vi "HAL-AI.vi"(7 "Name(\"\" to use uuid)":string="CSM-Module") -> ()   [LabVIEW 2020]
doc: "------------- lvcsm -------------\n[CSMStates]\nItem 0 = \"Idle\"\nItem 1 = \"CSM Documentation\"\nItem 2 = \"Error Handler\"\nItem 3 = \"VI Reference\"\nItem 4 = \"Critical Error\"\nItem 5 = \"Target Busy Error\"\nItem 6 = \"Target Timeout Error\"\nItem 7 = \"Target Error\"\nItem 8 = \"Async Response\"\nItem 9 = \"Response\"\nItem 10 = \"Async Message Posted\"\nItem 11 = \"Initialize Core Data\"\nItem 12 = \"Exit\"\nItem 13 = \"Data: Initialize\"\nItem 14 = \"Data: Get Configuration\"\nItem 15 = \"Data: Get Internal Data\"\nItem 16 = \"Data: Set Configuration\"\nItem 17 = \"Data: Update Indicators\"\nItem 18 = \"Data: Cleanup\"\nItem 19 = \"Macro: Initialize\"\nItem 20 = \"Macro: Exit\"\nItem 21 = \"Channels\"\nItem 22 = \"read\"\nItem 23 = \"read(massdata)\"\nItem 24 = \"read all\"\nItem 25 = \"DoSth: DoA\"\nItem 26 = \"DoSth: DoB\"\n\n[CSMStatus]\nItem 0 = \"Error Occurred@Error Handler\""
uses:
  4e85c3fb-ef85-4e26-a42c-c5beb394b70a.vi
  3806dceb-3f37-4f57-9f18-971811feca89.vi
  3ab58302-ba21-4fa6-a4e6-5e0190e36a76.vi
  c8f15f2d-01d5-4330-b5b0-2e0c665b45aa.vi
  a8188fcd-c635-40c0-88bb-da73c8fc0970.vi
  2d894bb3-d511-4c50-a434-1d8b5ddcf511.vi
  3a3714ae-08be-45b6-9f70-6e503687bd9b.vi
  0b2eaf5c-92e0-4609-89e4-060a3e7ae5c6.vi
  e9c7e813-d0b7-45e0-ac3a-d1de35bf1555.vi
  <userlib>/_NEVSTOP/Communicable State Machine(CSM)/_Support/Common/Format Timestamp.vi
  <userlib>/_NEVSTOP/Communicable State Machine(CSM)/AdvanceAPI/CSM - Revert Arguments-Safe String.vi
  <userlib>/_NEVSTOP/Communicable State Machine(CSM)/AdvanceAPI/CSM - Make String Arguments Safe.vi
  <userlib>/_NEVSTOP/Communicable State Machine(CSM)/AdvanceAPI/CSM - Break Down Multiple States String.vi
  <userlib>/_NEVSTOP/Communicable State Machine(CSM)/AdvanceAPI/CSM - Compact Multiple States.vi
  <userlib>/_NEVSTOP/Communicable State Machine(CSM)/AdvanceAPI/CSM - Keywords.vi
  <userlib>/_NEVSTOP/Communicable State Machine(CSM)/_Shared/Trim Single-line Text.vi
  <userlib>/_NEVSTOP/Communicable State Machine(CSM)/addons/API-String-Arugments-Support/_Support/Query Data as API String Arguments(variant).vi
  <userlib>/_NEVSTOP/Communicable State Machine(CSM)/addons/API-String-Arugments-Support/_Support/Convert API String Arguments to Data(variant).vi
  <userlib>/_NEVSTOP/Communicable State Machine(CSM)/addons/API-String-Arugments-Support/_Support/Data To API String Arguments.vi
  <userlib>/_NEVSTOP/Communicable State Machine(CSM)/addons/MassData-Parameter/_support/FGV-MassData(lvlibp).vi
  <userlib>/_NEVSTOP/Communicable State Machine(CSM)/Communicable State Machine.lvlib
panel:
  out "Error Occurred":errorcluster
  out "State History":string
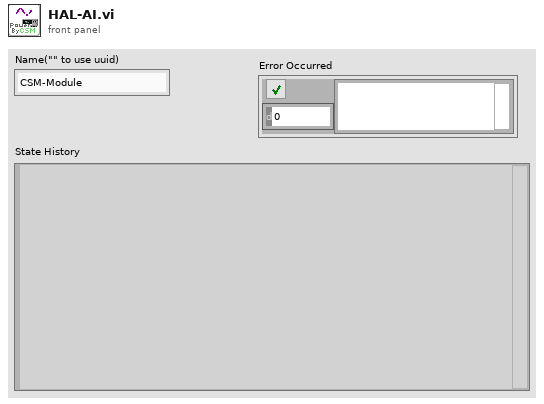
[diagram p1: front panel]
types:
  T1 = enum32{"Invalid", "Standard", "Closed", "Hidden", "Minimized", "Maximized"}
  T2 = enum32{"invalid app kind", "Development System", "Run Time System", "Student Edition", "Embedded LabVIEW", "Evaluation", "Custom"}
  T3 = typedef "Communicable State Machine.lvlib/_CSM_Response Source Message.ctl" = cluster{"‘State":string, "’Arguments":string, "’Error":errorcluster}
  T4 = cluster{"Current VI Reference":refnum<vi>, "Close Panel on Exit?":bool}
  T5 = cluster{"Core":cluster{"Current VI Reference":refnum<vi>, "Close Panel on Exit?":bool}, "Your Boolean data":bool, "Channels":string[]}
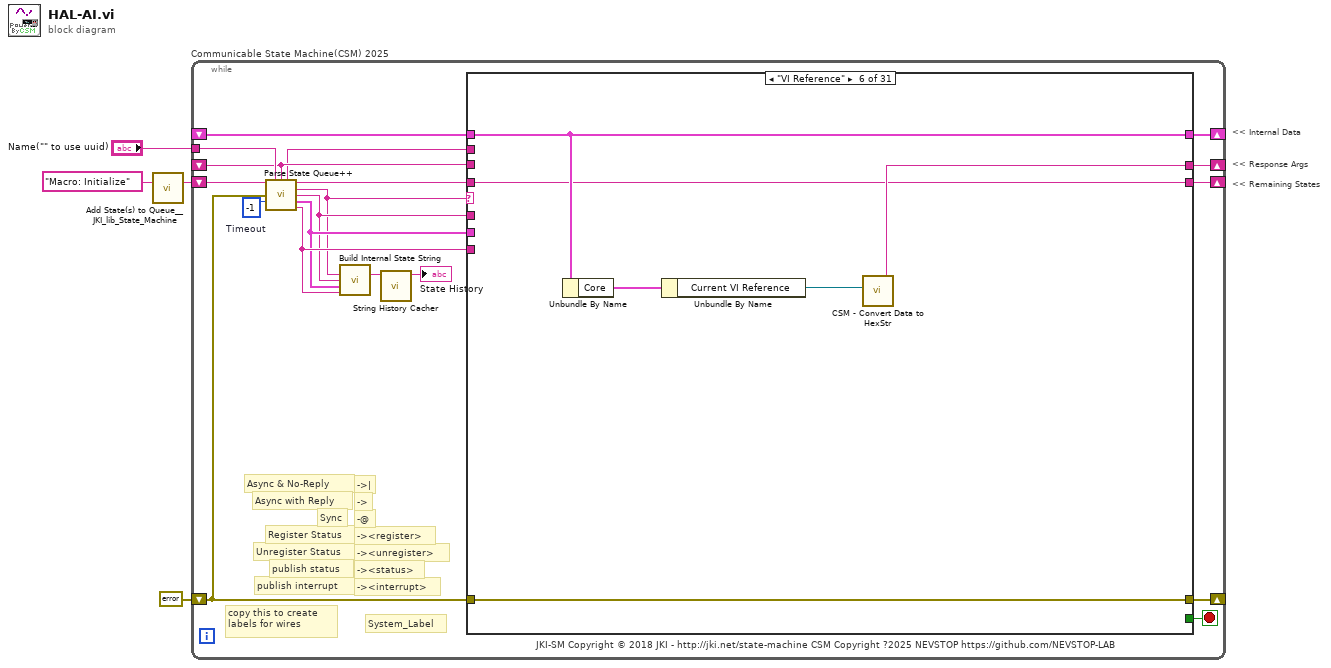
[diagram p0: block diagram]
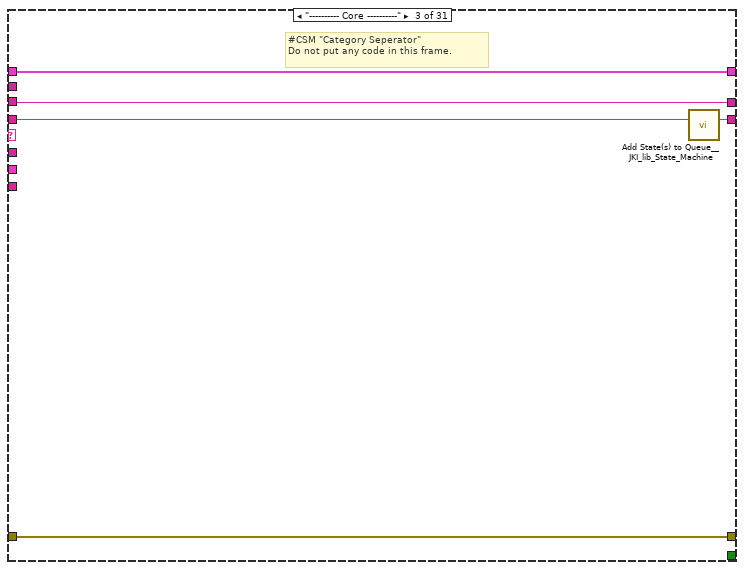
[diagram p4: hidden frame]
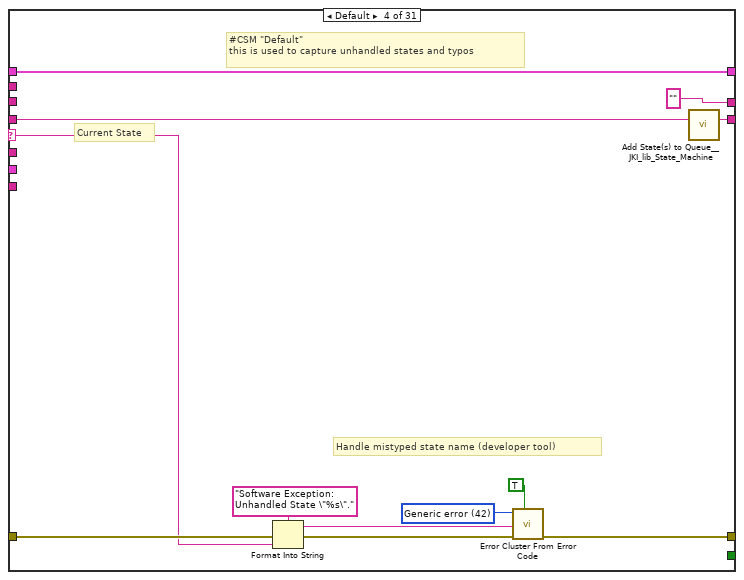
[diagram p5: hidden frame]
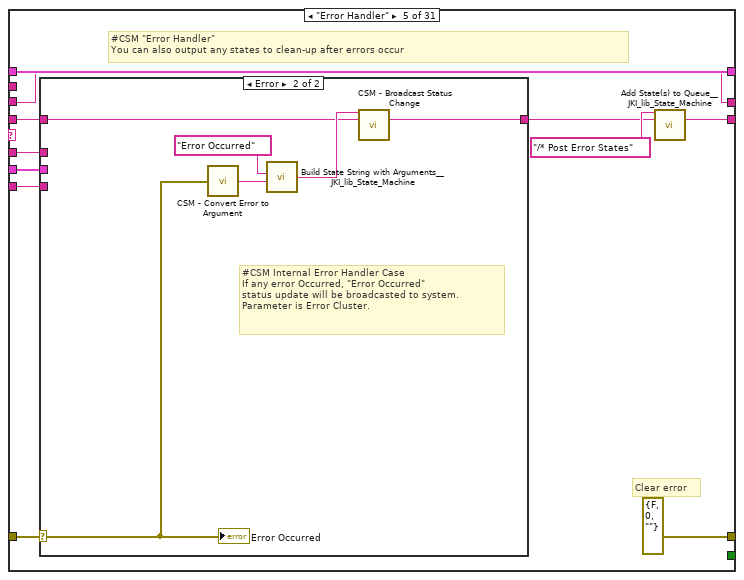
[diagram p6: hidden frame]
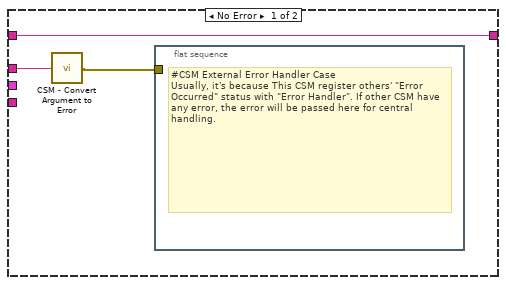
[diagram p7: hidden frame]
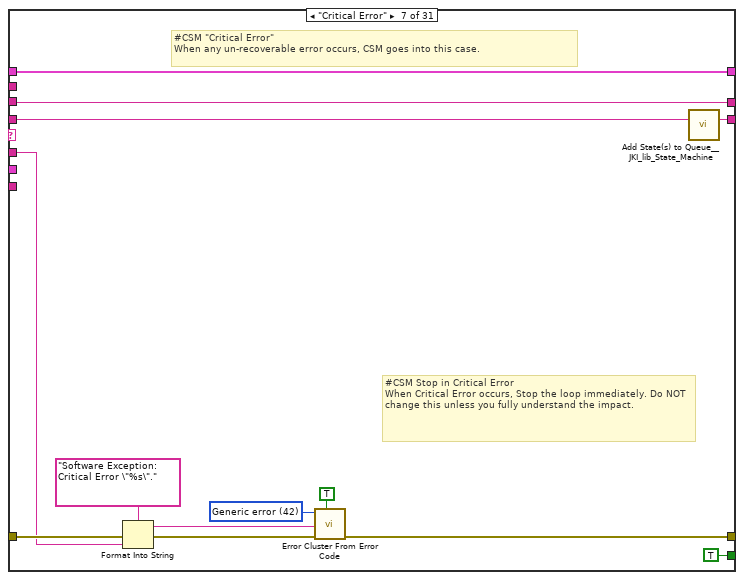
[diagram p8: hidden frame]
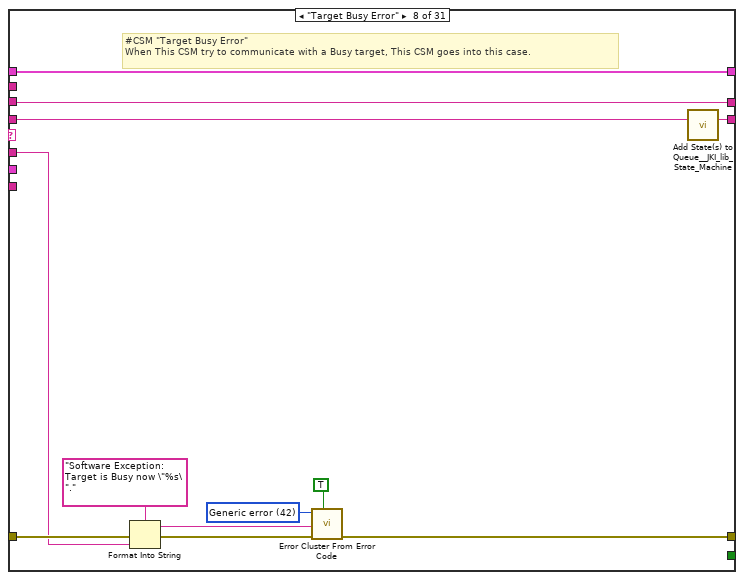
[diagram p9: hidden frame]
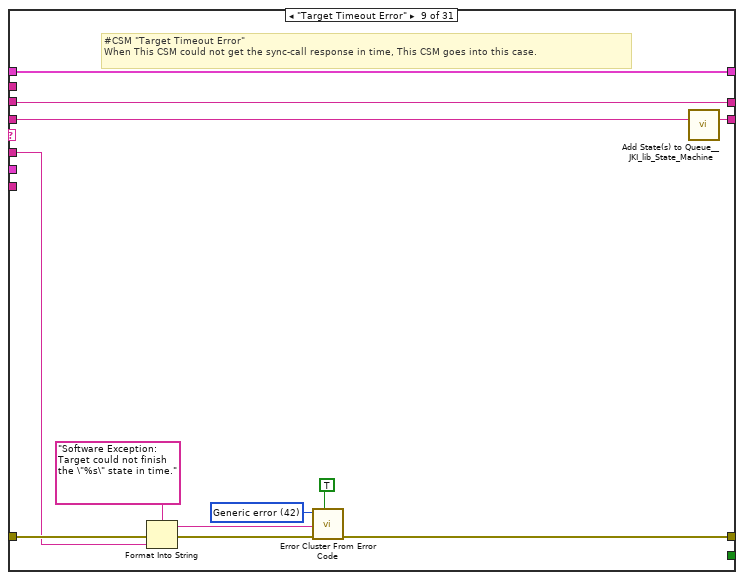
[diagram p10: hidden frame]
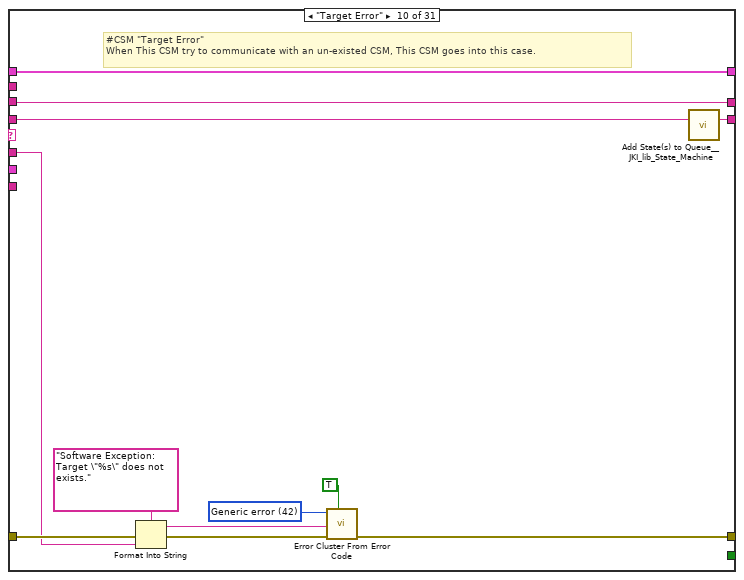
[diagram p11: hidden frame]
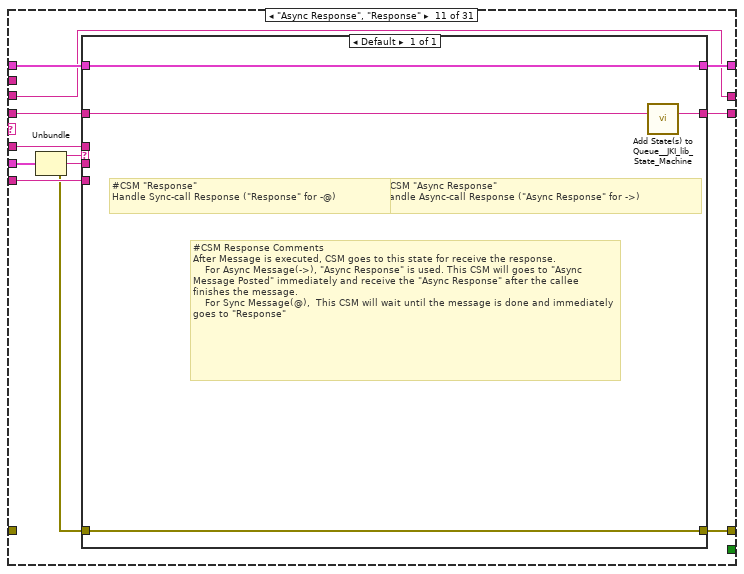
[diagram p12: hidden frame]
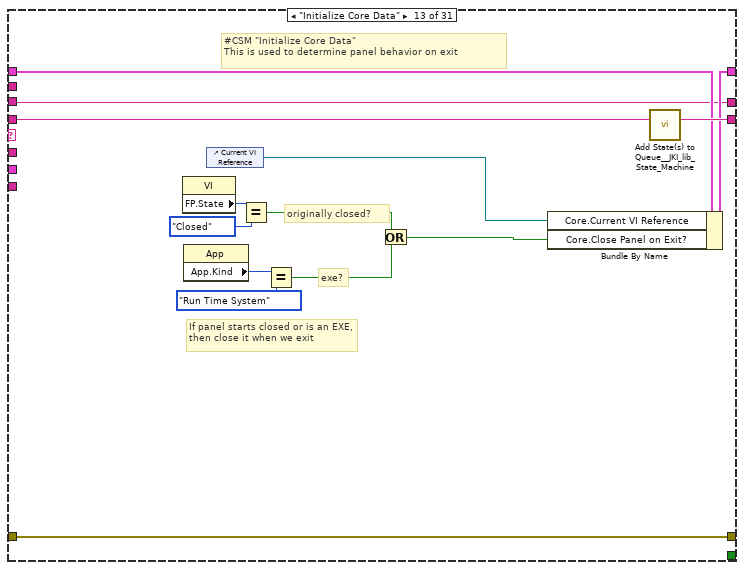
[diagram p14: hidden frame]
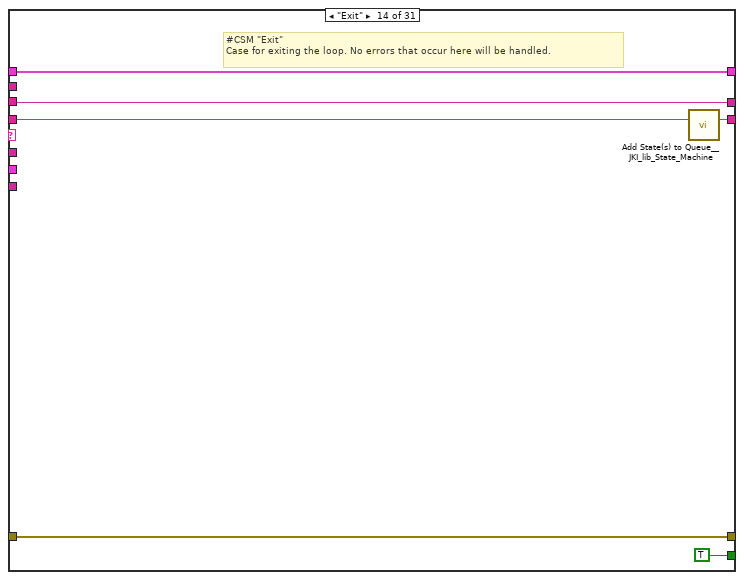
[diagram p15: hidden frame]
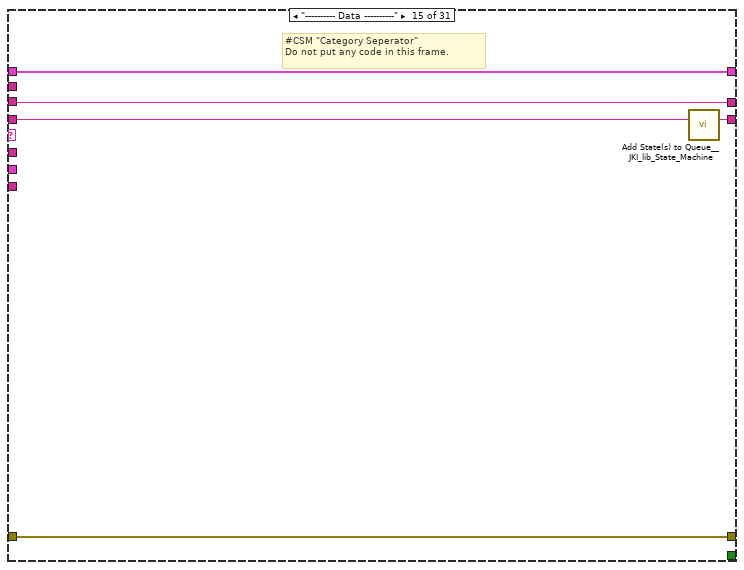
[diagram p16: hidden frame]
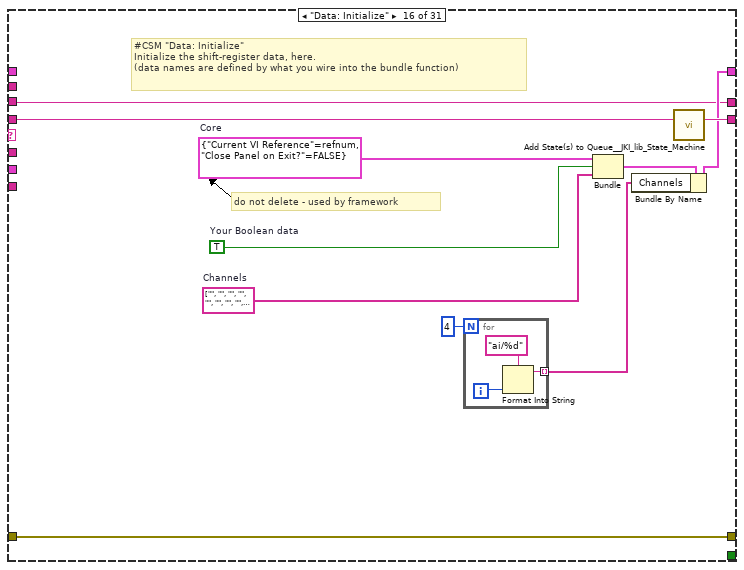
[diagram p17: hidden frame]
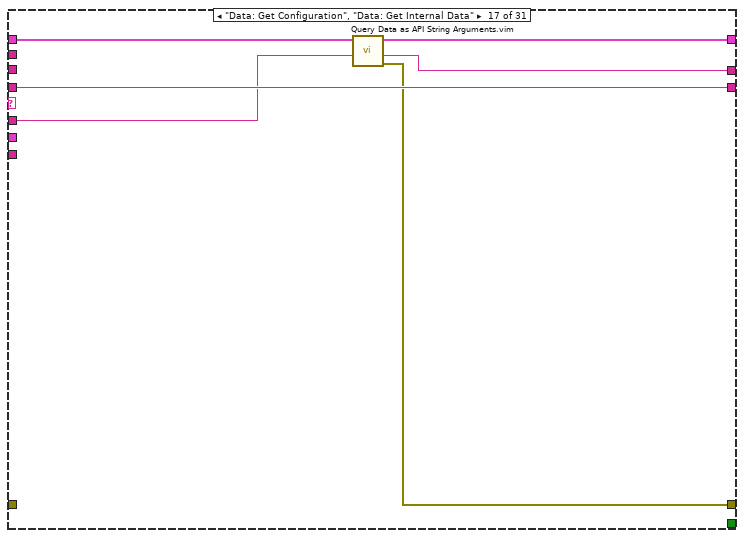
[diagram p18: hidden frame]
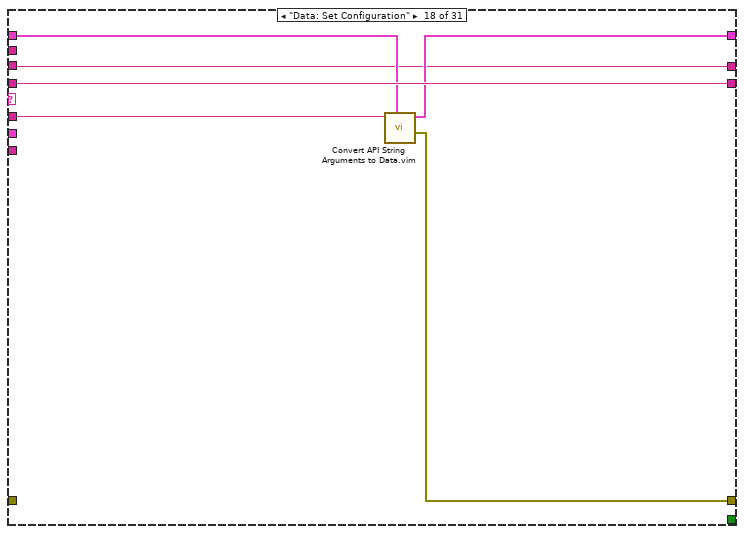
[diagram p19: hidden frame]
diagram:
  # "<< Internal Data"
  # "<< Response Args"
  # "<< Remaining States"
  n1 = call <vilib>:"Add State(s) to Queue__JKI_lib_State_Machine.vi"("State(s) in (\"\")"="Macro: Initialize" ("Init States(\"Macro: Initialize\")")) -> ("States Out"=w3:string)  [unwired: 14 in]
  n2 = while "Communicable State Machine(CSM) 2025" {
    shift-right: [w18] -> _
    shift-left: _ -> [w17]
    shift-right: [w21] -> _
    shift-left: errorcluster {"status"=FALSE, "code"=0, "source"=""} ("error out") -> [w5]
    shift-right: [w20] -> _
    shift-left: w3 -> [w22]
    tunnel: "Name(\"\" to use uuid)" -> [w14]
    shift-right: [w15] -> _
    shift-left: _ -> [w7]
    stop <- w19 stop-if-true
    w16 = -1  # Timeout
    # "copy this to create labels for wires"
    # "System_Label"
    # "-><interrupt>"
    # "-><status>"
    # "-><unregister>"
    # "-><register>"
    # "-@"
    # "->"
    # "->|"
    # "publish interrupt"
    # "publish status"
    # "Unregister Status"
    # "Register Status"
    # "Sync"
    # "Async with Reply"
    # "Async & No-Reply"
    # "JKI-SM Copyright © 2018 JKI - http://jki.net/state-machine CSM Copyright ?2025 NEVSTOP https://github.com/NEVSTOP-LAB"
    n3 = call <userlib>:"Parse State Queue++.vi"("State Queue"=w22, "Name (\"\" to Use UUID)"=w14, "Response Arguments"=w7, "Previous Error"=w5, "Dequeue (1 ms)"=w16) -> ("Name Used"=w6:string, "Remaining States"=w23:string, "Current State"=w8:string, "Arguments"=w9:string, "Additional Information"=w10:T3, "Source CSM"=w11:string)  [unwired: 5 in]
    n4 = call <userlib>:"Build Internal State String.vi"("State"=w8, "Arguments (\"\")"=w9, "Additional Information"=w10, "Source (\"\")"=w11) -> ("State With Arguments"=w12:string)  [unwired: 11 in]
    n5 = call <userlib>:"String History Cacher.vi"("String"=w12) -> ("String Cache"=→"State History":string)  [unwired: 10 in]
    n6 = case shown="\"VI Reference\"" w8 {
      selector: w8 -> [_ _ _ w38 _ _ _ _ _ _ _ _ _ _ _ _ _ _ _ _ _ _ _ _ _ _ _ _ _ _ _]
      tunnel: w23 -> [w25 w30 w36 w42 w53 w70 w81 w94 w106 w118 w129 w142 w157 w163 w168 w179 w188 w194 w197 w205 w210 w216 w222 w225 w230 w250 w273 w291 w300 w305 w310]
      tunnel: w9 -> [_ _ _ _ w52 _ w77 w90 w102 w114 w128 _ _ _ _ _ w183 w193 _ _ _ _ _ _ _ w249 w272 w290 _ _ _]
      tunnel: w17 -> [w26 w29 w33 w40 w58 w74 w79 w92 w104 w116 w130 w141 w150 w161 w165 _ w187 w192 w196 w200 w207 w213 w219 w224 w227 w244 w267 w285 w297 w302 w307]
      tunnel: [w27 w31 w34 w44 errorcluster {"status"=FALSE, "code"=0, "source"=""} ("error out") w69 w83 w89 w101 w113 w133 w143 w154 w160 w166 w176 w184 w190 w198 w201 w208 w214 w220 w226 w231 w237 w260 w292 w298 w303 w308] -> w21
      tunnel: w5 -> [w27 w31 w34 w43 w56 w69 w82 w95 w107 w119 _ w143 w154 w160 w166 w176 _ _ w198 w202 w208 w214 w220 w226 w231 _ _ w292 w298 w303 w308]
      tunnel: [w25 w30 w35 w41 w54 w70 w80 w93 w105 w117 w131 w142 w156 w162 w167 w178 w188 w194 w197 w204 w209 w215 w221 w225 w230 w250 w273 w291 w299 w304 w309] -> w20
      tunnel: [_ _ _ _ _ _ TRUE _ _ _ _ _ _ TRUE _ _ _ _ _ _ _ _ _ _ _ _ _ _ _ _ _] -> w19
      tunnel: [w26 w29 w33 w40 w58 w74 w79 w92 w104 w116 w132 w141 w155 w161 w165 w172 w186 w191 w196 w200 w207 w213 w219 w224 w227 w244 w267 w285 w297 w302 w307] -> w18
      tunnel: w11 -> [_ _ _ _ w51 _ _ _ _ _ w126 _ _ _ _ _ _ _ _ _ _ _ _ _ _ _ _ _ _ _ _]
      tunnel: w10 -> [_ _ _ _ w50 _ _ _ _ _ w127 _ _ _ _ _ _ _ _ _ _ _ _ _ _ _ _ _ _ _ _]
      tunnel: [w24 w28 w32 "" w49 w71 w75 w88 w100 w112 w124 w140 w144 w158 w164 w169 w185 w189 w195 w199 w206 w211 w217 w223 w228 w245 w268 w288 w296 "DoA Finished" "DoB Finished"] -> w15
      tunnel: w6 -> [_ _ _ _ _ _ _ _ _ _ _ _ _ _ _ _ _ _ _ _ _ _ _ _ _ _ _ _ _ _ _]
      tunnel: w7 -> [w24 w28 w32 _ w49 _ w75 w88 w100 w112 w124 w140 w144 w158 w164 w169 _ w189 w195 w199 w206 w211 w217 w223 _ _ _ _ w296 _ _]
      frame "", "Idle" {
        # "#CSM \"Idle/Event Handler\"\nexecutes when the state queue is empty"
      }
      frame "CSM Documentation" {
        # "CSM Documentation"
        # "#CSM Commenting\nTo add a comment use \"//\" or \"#\" and all text to the right will be ignored\n\nCommenting Example:\nUI: Initialize // This initializes the UI\n// Another comment line"
        # "#CSM State Syntax\n\n    // Local Message Example\n    DoSth: DoA >> Arguments\n\n    // Sync Call Example\n    API: xxxx >> Arguments -@ TargetModule\n\n    // Async Call Example\n    API: xxxx >> Arguments -> TargetModule\n\n    // Async Call without Reply Example\n    API: xxxx >> Arguments ->| TargetModule\n\n    // Broadcast normal status:\n    Status >> StatusArguments  -><status>\n\n    // Broadcast Interrupt status:\n    Interrupt >> StatusArguments  -><interrupt>\n\n    // Register Source Module's status to Handler Module\n    Status@Source Module >> Handler Module@Handler Module -><register>\n\n    // Unegister Source Module's status\n    Status@Source Module >> Handler Module -><unregister>"
        # "#CSM README FIRST\n\nCSM is a LabVIEW application framework that builds upon JKI State Machine (CSM). It follows the pattern of CSM and extends the keywords to describe message communication between CSM modules, including concepts such as Sync-Message, Async-Message, Subscription/Unsubscription of status - essential elements for creating reusable code modules. For more information, please visit the CSM wiki: https://github.com/NEVSTOP-LAB/JKI-State-Machine-Plus-Plus/wiki\n\nFor instructions on JKI State Machine, visit: http://jki.net/state-machine/\nFor information about CSM, visit: https://github.com/NEVSTOP-LAB"
        # "#CSM \"Documentation\"\nCase for holding CSM Documenation"
      }
      frame "---------- Core ----------" {
        # "#CSM \"Category Seperator\"\nDo not put any code in this frame."
        n7 = call <vilib>:"Add State(s) to Queue__JKI_lib_State_Machine.vi"("State(s) in (\"\")"=w36) -> ("States Out"=w35:string)  [unwired: 14 in]
      }
      frame Default {
        w47 = 42 items=["No error", "Argument error", "Memory is full", "Out of zone", "End of file", "File already open", "Generic file I/O error", "File not found", "File permission error", "Disk is full", "Duplicate path", "Too many files open", "System feature not enabled", "Resource file not found", "Cannot add resource", "Resource not found", "Image not found", "Image memory error", "Pen does not exist", "Config type invalid", "Config token not found", "Config parse error", "Config memory error", "Bad external code format", "Bad external code offset", "External code not present", "Null window", "Destroy window error", "Null menu", "Print aborted", "Bad print record", "Print driver error", "Windows error during printing", "Memory error during printing", "Print dialog error", "Generic print error", "Invalid device refnum", "Device not found", "Device parameter error", "Device unit error", "Cannot open device", "Device call aborted", "Generic error", "Cancelled by user", "Object ID too low", "Object ID too high", "Object not in heap", "Unknown heap", "Unknown object (invalid DefProc)", "Unknown object (DefProc not in table)", "Message out of range", "Invalid (null) method", "Unknown message", "Manager call not supported", "Bad address", "Network operation in progress", "Network operation timed out", "Connection is busy", "Network attribute not supported", "Network error", "Address in use", "System out of memory", "Connection aborted", "Connection refused", "Not connected", "Already connected", "Connection closed", "Initialization error (interapplication manager)", "Bad occurrence", "Wait on unbound occurrence handler", "Occurrence queue overflow", "Datalog type conflict", "Unused", "Unrecognized type (interapplication manager)", "Memory corrupt", "Failed to make temporary DLL", "Old CIN version", "Drag socket not found", "Failed to load drop-object", "Failed to register OLE object", "Failed to release OLE object", "Format specifier type mismatch", "Unknown format specifier", "Too few format specifiers", "Too many format specifiers", "Scan failed", "Newer CIN version", "Error converting to variant", "Runtime menu error", "Password tampered", "Variant attribute not found", "Incompatible variant data type", "Event data is not available", "Event Store is not present", "Occurrence is not found", "Event Queue is not created", "Event info is not available", "Refnum passed is NULL", "Error retrieving Class GUID", "Error retrieving CoClass GUID", "Error retrieving TypeLib GUID.", "Bad built application magic bytes.", "Specific driver is different from the specific driver associated with the Logical Name.", "There is no session opened to the class driver.", "Max Error", "MAX - Error with config objects", "MAX - Error loading configuration", "MAX - Group not supported"]
        # "#CSM \"Default\"\nthis is used to capture unhandled states and typos"
        # "Current State"
        # "Handle mistyped state name (developer tool)"
        n8 = Format Into String(format string="Software Exception: Unhandled State \"%s\"." ("message"), error in=w43, w38) -> (resulting string=w46:string, error out=w45:errorcluster)  [unwired: 1 in]
        n9 = call <vilib>:"Error Cluster From Error Code.vi"("show call chain? (False)"=TRUE, "error in (no error)"=w45, "error message (\"\")"=w46, "error code (0)"=w47) -> ("error out"=w44:errorcluster)  [unwired: 5 in]
        n10 = call <vilib>:"Add State(s) to Queue__JKI_lib_State_Machine.vi"("State(s) in (\"\")"=w42) -> ("States Out"=w41:string)  [unwired: 14 in]
      }
      frame "Error Handler" {
        # "#CSM \"Error Handler\"\nYou can also output any states to clean-up after errors occur"
        # "Clear error"
        n11 = case shown="Error" w56 {
          selector: w56 -> [_ w63]
          tunnel: [w62 w65] -> w55
          tunnel: w53 -> [w62 w64]
          tunnel: w52 -> [w61 _]
          tunnel: w51 -> [_ _]
          tunnel: w50 -> [_ _]
          frame No Error {
            n12 = call <userlib>:"CSM - Convert Argument to Error.vi"("Argument"=w61) -> ("Error"=w60:errorcluster)  [unwired: 4 in]
            n13 = flat-sequence {
              tunnel: w60 -> [_]
              frame #0 {
                # "#CSM External Error Handler Case\nUsually, it's because This CSM register others' \"Error Occurred\" status with \"Error Handler\". If other CSM have any error, the error will be passed here for central handling."
              }
            }
          }
          frame Error {
            # "#CSM Internal Error Handler Case \nIf any error Occurred, \"Error Occurred\" \nstatus update will be broadcasted to system.\nParameter is Error Cluster."
            n14 = call <userlib>:"CSM - Convert Error to Argument.vi"("Error"=w63) -> ("Argument"=w67:string)  [unwired: 4 in]
            n15 = call <vilib>:"Build State String with Arguments__JKI_lib_State_Machine.vi"("Arguments (\"\")"=w67, "State"="Error Occurred" ("Status with Arguments")) -> ("State with Arguments"=w66:string)  [unwired: 4 in]
            n16 = call <userlib>:"CSM - Broadcast Status Change.vi"("Status With Arguments"=w66, "State Queue"=w64) -> ("Remaining States"=w65:string)  [unwired: 13 in]
            "Error Occurred" <- w63
          }
        }
        n17 = call <vilib>:"Add State(s) to Queue__JKI_lib_State_Machine.vi"("State(s) in Front (\"\")"="/* Post Error States", "State(s) in (\"\")"=w55) -> ("States Out"=w54:string)  [unwired: 13 in]
      }
      frame "VI Reference" {
        n18 = Unbundle By Name(w74) -> ("Core"=w73:T4)
        n19 = Unbundle By Name(w73) -> ("Current VI Reference"=w72:refnum<vi>)
        n20 = call <userlib>:"CSM - Convert Data to HexStr.vi"("Variant"=w72) -> ("HEX String (0-9,A-F)"=w71:string)  [unwired: 8 in]
      }
      frame "Critical Error" {
        w86 = 42 items=["No error", "Argument error", "Memory is full", "Out of zone", "End of file", "File already open", "Generic file I/O error", "File not found", "File permission error", "Disk is full", "Duplicate path", "Too many files open", "System feature not enabled", "Resource file not found", "Cannot add resource", "Resource not found", "Image not found", "Image memory error", "Pen does not exist", "Config type invalid", "Config token not found", "Config parse error", "Config memory error", "Bad external code format", "Bad external code offset", "External code not present", "Null window", "Destroy window error", "Null menu", "Print aborted", "Bad print record", "Print driver error", "Windows error during printing", "Memory error during printing", "Print dialog error", "Generic print error", "Invalid device refnum", "Device not found", "Device parameter error", "Device unit error", "Cannot open device", "Device call aborted", "Generic error", "Cancelled by user", "Object ID too low", "Object ID too high", "Object not in heap", "Unknown heap", "Unknown object (invalid DefProc)", "Unknown object (DefProc not in table)", "Message out of range", "Invalid (null) method", "Unknown message", "Manager call not supported", "Bad address", "Network operation in progress", "Network operation timed out", "Connection is busy", "Network attribute not supported", "Network error", "Address in use", "System out of memory", "Connection aborted", "Connection refused", "Not connected", "Already connected", "Connection closed", "Initialization error (interapplication manager)", "Bad occurrence", "Wait on unbound occurrence handler", "Occurrence queue overflow", "Datalog type conflict", "Unused", "Unrecognized type (interapplication manager)", "Memory corrupt", "Failed to make temporary DLL", "Old CIN version", "Drag socket not found", "Failed to load drop-object", "Failed to register OLE object", "Failed to release OLE object", "Format specifier type mismatch", "Unknown format specifier", "Too few format specifiers", "Too many format specifiers", "Scan failed", "Newer CIN version", "Error converting to variant", "Runtime menu error", "Password tampered", "Variant attribute not found", "Incompatible variant data type", "Event data is not available", "Event Store is not present", "Occurrence is not found", "Event Queue is not created", "Event info is not available", "Refnum passed is NULL", "Error retrieving Class GUID", "Error retrieving CoClass GUID", "Error retrieving TypeLib GUID.", "Bad built application magic bytes.", "Specific driver is different from the specific driver associated with the Logical Name.", "There is no session opened to the class driver.", "Max Error", "MAX - Error with config objects", "MAX - Error loading configuration", "MAX - Group not supported"]
        # "#CSM \"Critical Error\"\nWhen any un-recoverable error occurs, CSM goes into this case."
        # "#CSM Stop in Critical Error\nWhen Critical Error occurs, Stop the loop immediately. Do NOT change this unless you fully understand the impact."
        n21 = Format Into String(format string="Software Exception: Critical Error \"%s\"." ("message"), error in=w82, w77) -> (resulting string=w85:string, error out=w84:errorcluster)  [unwired: 1 in]
        n22 = call <vilib>:"Error Cluster From Error Code.vi"("show call chain? (False)"=TRUE, "error in (no error)"=w84, "error message (\"\")"=w85, "error code (0)"=w86) -> ("error out"=w83:errorcluster)  [unwired: 5 in]
        n23 = call <vilib>:"Add State(s) to Queue__JKI_lib_State_Machine.vi"("State(s) in (\"\")"=w81) -> ("States Out"=w80:string)  [unwired: 14 in]
      }
      frame "Target Busy Error" {
        w98 = 42 items=["No error", "Argument error", "Memory is full", "Out of zone", "End of file", "File already open", "Generic file I/O error", "File not found", "File permission error", "Disk is full", "Duplicate path", "Too many files open", "System feature not enabled", "Resource file not found", "Cannot add resource", "Resource not found", "Image not found", "Image memory error", "Pen does not exist", "Config type invalid", "Config token not found", "Config parse error", "Config memory error", "Bad external code format", "Bad external code offset", "External code not present", "Null window", "Destroy window error", "Null menu", "Print aborted", "Bad print record", "Print driver error", "Windows error during printing", "Memory error during printing", "Print dialog error", "Generic print error", "Invalid device refnum", "Device not found", "Device parameter error", "Device unit error", "Cannot open device", "Device call aborted", "Generic error", "Cancelled by user", "Object ID too low", "Object ID too high", "Object not in heap", "Unknown heap", "Unknown object (invalid DefProc)", "Unknown object (DefProc not in table)", "Message out of range", "Invalid (null) method", "Unknown message", "Manager call not supported", "Bad address", "Network operation in progress", "Network operation timed out", "Connection is busy", "Network attribute not supported", "Network error", "Address in use", "System out of memory", "Connection aborted", "Connection refused", "Not connected", "Already connected", "Connection closed", "Initialization error (interapplication manager)", "Bad occurrence", "Wait on unbound occurrence handler", "Occurrence queue overflow", "Datalog type conflict", "Unused", "Unrecognized type (interapplication manager)", "Memory corrupt", "Failed to make temporary DLL", "Old CIN version", "Drag socket not found", "Failed to load drop-object", "Failed to register OLE object", "Failed to release OLE object", "Format specifier type mismatch", "Unknown format specifier", "Too few format specifiers", "Too many format specifiers", "Scan failed", "Newer CIN version", "Error converting to variant", "Runtime menu error", "Password tampered", "Variant attribute not found", "Incompatible variant data type", "Event data is not available", "Event Store is not present", "Occurrence is not found", "Event Queue is not created", "Event info is not available", "Refnum passed is NULL", "Error retrieving Class GUID", "Error retrieving CoClass GUID", "Error retrieving TypeLib GUID.", "Bad built application magic bytes.", "Specific driver is different from the specific driver associated with the Logical Name.", "There is no session opened to the class driver.", "Max Error", "MAX - Error with config objects", "MAX - Error loading configuration", "MAX - Group not supported"]
        # "#CSM \"Target Busy Error\"\nWhen This CSM try to communicate with a Busy target, This CSM goes into this case."
        n24 = Format Into String(format string="Software Exception: Target is Busy now \"%s\"." ("message"), error in=w95, w90) -> (resulting string=w97:string, error out=w96:errorcluster)  [unwired: 1 in]
        n25 = call <vilib>:"Error Cluster From Error Code.vi"("show call chain? (False)"=TRUE, "error in (no error)"=w96, "error message (\"\")"=w97, "error code (0)"=w98) -> ("error out"=w89:errorcluster)  [unwired: 5 in]
        n26 = call <vilib>:"Add State(s) to Queue__JKI_lib_State_Machine.vi"("State(s) in (\"\")"=w94) -> ("States Out"=w93:string)  [unwired: 14 in]
      }
      frame "Target Timeout Error" {
        w110 = 42 items=["No error", "Argument error", "Memory is full", "Out of zone", "End of file", "File already open", "Generic file I/O error", "File not found", "File permission error", "Disk is full", "Duplicate path", "Too many files open", "System feature not enabled", "Resource file not found", "Cannot add resource", "Resource not found", "Image not found", "Image memory error", "Pen does not exist", "Config type invalid", "Config token not found", "Config parse error", "Config memory error", "Bad external code format", "Bad external code offset", "External code not present", "Null window", "Destroy window error", "Null menu", "Print aborted", "Bad print record", "Print driver error", "Windows error during printing", "Memory error during printing", "Print dialog error", "Generic print error", "Invalid device refnum", "Device not found", "Device parameter error", "Device unit error", "Cannot open device", "Device call aborted", "Generic error", "Cancelled by user", "Object ID too low", "Object ID too high", "Object not in heap", "Unknown heap", "Unknown object (invalid DefProc)", "Unknown object (DefProc not in table)", "Message out of range", "Invalid (null) method", "Unknown message", "Manager call not supported", "Bad address", "Network operation in progress", "Network operation timed out", "Connection is busy", "Network attribute not supported", "Network error", "Address in use", "System out of memory", "Connection aborted", "Connection refused", "Not connected", "Already connected", "Connection closed", "Initialization error (interapplication manager)", "Bad occurrence", "Wait on unbound occurrence handler", "Occurrence queue overflow", "Datalog type conflict", "Unused", "Unrecognized type (interapplication manager)", "Memory corrupt", "Failed to make temporary DLL", "Old CIN version", "Drag socket not found", "Failed to load drop-object", "Failed to register OLE object", "Failed to release OLE object", "Format specifier type mismatch", "Unknown format specifier", "Too few format specifiers", "Too many format specifiers", "Scan failed", "Newer CIN version", "Error converting to variant", "Runtime menu error", "Password tampered", "Variant attribute not found", "Incompatible variant data type", "Event data is not available", "Event Store is not present", "Occurrence is not found", "Event Queue is not created", "Event info is not available", "Refnum passed is NULL", "Error retrieving Class GUID", "Error retrieving CoClass GUID", "Error retrieving TypeLib GUID.", "Bad built application magic bytes.", "Specific driver is different from the specific driver associated with the Logical Name.", "There is no session opened to the class driver.", "Max Error", "MAX - Error with config objects", "MAX - Error loading configuration", "MAX - Group not supported"]
        # "#CSM \"Target Timeout Error\"\nWhen This CSM could not get the sync-call response in time, This CSM goes into this case."
        n27 = Format Into String(format string="Software Exception: Target could not finish the \"%s\" state in time." ("message"), error in=w107, w102) -> (resulting string=w109:string, error out=w108:errorcluster)  [unwired: 1 in]
        n28 = call <vilib>:"Error Cluster From Error Code.vi"("show call chain? (False)"=TRUE, "error in (no error)"=w108, "error message (\"\")"=w109, "error code (0)"=w110) -> ("error out"=w101:errorcluster)  [unwired: 5 in]
        n29 = call <vilib>:"Add State(s) to Queue__JKI_lib_State_Machine.vi"("State(s) in (\"\")"=w106) -> ("States Out"=w105:string)  [unwired: 14 in]
      }
      frame "Target Error" {
        w122 = 42 items=["No error", "Argument error", "Memory is full", "Out of zone", "End of file", "File already open", "Generic file I/O error", "File not found", "File permission error", "Disk is full", "Duplicate path", "Too many files open", "System feature not enabled", "Resource file not found", "Cannot add resource", "Resource not found", "Image not found", "Image memory error", "Pen does not exist", "Config type invalid", "Config token not found", "Config parse error", "Config memory error", "Bad external code format", "Bad external code offset", "External code not present", "Null window", "Destroy window error", "Null menu", "Print aborted", "Bad print record", "Print driver error", "Windows error during printing", "Memory error during printing", "Print dialog error", "Generic print error", "Invalid device refnum", "Device not found", "Device parameter error", "Device unit error", "Cannot open device", "Device call aborted", "Generic error", "Cancelled by user", "Object ID too low", "Object ID too high", "Object not in heap", "Unknown heap", "Unknown object (invalid DefProc)", "Unknown object (DefProc not in table)", "Message out of range", "Invalid (null) method", "Unknown message", "Manager call not supported", "Bad address", "Network operation in progress", "Network operation timed out", "Connection is busy", "Network attribute not supported", "Network error", "Address in use", "System out of memory", "Connection aborted", "Connection refused", "Not connected", "Already connected", "Connection closed", "Initialization error (interapplication manager)", "Bad occurrence", "Wait on unbound occurrence handler", "Occurrence queue overflow", "Datalog type conflict", "Unused", "Unrecognized type (interapplication manager)", "Memory corrupt", "Failed to make temporary DLL", "Old CIN version", "Drag socket not found", "Failed to load drop-object", "Failed to register OLE object", "Failed to release OLE object", "Format specifier type mismatch", "Unknown format specifier", "Too few format specifiers", "Too many format specifiers", "Scan failed", "Newer CIN version", "Error converting to variant", "Runtime menu error", "Password tampered", "Variant attribute not found", "Incompatible variant data type", "Event data is not available", "Event Store is not present", "Occurrence is not found", "Event Queue is not created", "Event info is not available", "Refnum passed is NULL", "Error retrieving Class GUID", "Error retrieving CoClass GUID", "Error retrieving TypeLib GUID.", "Bad built application magic bytes.", "Specific driver is different from the specific driver associated with the Logical Name.", "There is no session opened to the class driver.", "Max Error", "MAX - Error with config objects", "MAX - Error loading configuration", "MAX - Group not supported"]
        # "#CSM \"Target Error\"\nWhen This CSM try to communicate with an un-existed CSM, This CSM goes into this case."
        n30 = Format Into String(format string="Software Exception: Target \"%s\" does not exists." ("message"), error in=w119, w114) -> (resulting string=w121:string, error out=w120:errorcluster)  [unwired: 1 in]
        n31 = call <vilib>:"Error Cluster From Error Code.vi"("show call chain? (False)"=TRUE, "error in (no error)"=w120, "error message (\"\")"=w121, "error code (0)"=w122) -> ("error out"=w113:errorcluster)  [unwired: 5 in]
        n32 = call <vilib>:"Add State(s) to Queue__JKI_lib_State_Machine.vi"("State(s) in (\"\")"=w118) -> ("States Out"=w117:string)  [unwired: 14 in]
      }
      frame "Async Response", "Response" {
        n33 = Unbundle(w127) -> ("‘State"=w135:string, "’Arguments"=w134:string, "’Error"=w125:errorcluster)
        n34 = case shown="Default" w135 {
          tunnel: [w136] -> w131
          tunnel: w129 -> [w137]
          tunnel: [w139] -> w132
          tunnel: w130 -> [w139]
          tunnel: [w138] -> w133
          tunnel: w125 -> [w138]
          tunnel: w126 -> [_]
          tunnel: w128 -> [_]
          tunnel: w134 -> [_]
          frame Default {
            # "#CSM \"Async Response\"\nHandle Async-call Response (\"Async Response\" for ->)"
            # "#CSM \"Response\"\nHandle Sync-call Response (\"Response\" for -@)"
            # "#CSM Response Comments\nAfter Message is executed, CSM goes to this state for receive the response.\n    For Async Message(->), \"Async Response\" is used. This CSM will goes to \"Async Message Posted\" immediately and receive the \"Async Response\" after the callee finishes the message.\n    For Sync Message(@),  This CSM will wait until the message is done and immediately goes to \"Response\""
            n35 = call <vilib>:"Add State(s) to Queue__JKI_lib_State_Machine.vi"("State(s) in (\"\")"=w137) -> ("States Out"=w136:string)  [unwired: 14 in]
          }
        }
      }
      frame "Async Message Posted" {
        # "#CSM \"Async Message Posted\"\nAfter Async Message is posted (-> or ->| ), CSM goes to this state for post-action.\nYou can use Argument - State to tell which Async Message is called."
      }
      frame "Initialize Core Data" {
        # "#CSM \"Initialize Core Data\"\nThis is used to determine panel behavior on exit"
        # "originally closed?"
        # "exe?"
        # "If panel starts closed or is an EXE, then close it when we exit"
        n36 = property class="VI"() -> ("FP.State"=w147:T1)  [unwired: 2 in, 2 out]
        n37 = property class="App"() -> ("App.Kind"=w153:T2)  [unwired: 2 in, 2 out]
        n38 = control-ref of="Current VI Reference"() -> (w148:refnum<vi>)
        n39 = Equal?(x=w147, y=T1."Closed" ("Front Panel Window:State")) -> (x = y?=w145:bool)
        n40 = Equal?(x=w153, y=T2."Run Time System" ("Application:Kind")) -> (x = y?=w151:bool)
        n41 = Or(x=w145, y=w151) -> (x .or. y?=w149:bool)
        n42 = Bundle By Name(cluster=w150, "Core.Current VI Reference"=w148, "Core.Close Panel on Exit?"=w149) -> (w155:T5)
        n43 = call <vilib>:"Add State(s) to Queue__JKI_lib_State_Machine.vi"("State(s) in (\"\")"=w157) -> ("States Out"=w156:string)  [unwired: 14 in]
      }
      frame "Exit" {
        # "#CSM \"Exit\"\nCase for exiting the loop. No errors that occur here will be handled."
        n44 = call <vilib>:"Add State(s) to Queue__JKI_lib_State_Machine.vi"("State(s) in (\"\")"=w163) -> ("States Out"=w162:string)  [unwired: 14 in]
      }
      frame "---------- Data ----------" {
        # "#CSM \"Category Seperator\"\nDo not put any code in this frame."
        n45 = call <vilib>:"Add State(s) to Queue__JKI_lib_State_Machine.vi"("State(s) in (\"\")"=w168) -> ("States Out"=w167:string)  [unwired: 14 in]
      }
      frame "Data: Initialize" {
        w173 = string[] ["", "", "", "", "", "", "", "", ""]  # Channels
        w174 = T4 {"Current VI Reference"=refnum, "Close Panel on Exit?"=FALSE}  # Core
        w175 = TRUE  # Your Boolean data
        # "#CSM \"Data: Initialize\"\nInitialize the shift-register data, here.\n(data names are defined by what you wire into the bundle function)"
        # "do not delete - used by framework"
        n46 = for {
          N: 4 -> [_]
          tunnel: [w180] -> w171 mode=indexing
          i -> [w182]
          n47 = Format Into String(format string="ai/%d", w182) -> (resulting string=w180:string)  [unwired: 2 in, 1 out]
        }
        n48 = Bundle("Core"=w174, "Your Boolean data"=w175, "Channels"=w173) -> (w177:T5)  [unwired: 1 in]
        n49 = Bundle By Name(cluster=w177, "Channels"=w171) -> (w172:T5)
        n50 = call <vilib>:"Add State(s) to Queue__JKI_lib_State_Machine.vi"("State(s) in (\"\")"=w179) -> ("States Out"=w178:string)  [unwired: 14 in]
      }
      frame "Data: Get Configuration", "Data: Get Internal Data" {
        n51 = call "Query Data as API String Arguments.vim"("Name"=w183, "Cluster Data"=w187) -> ("error"=w184:errorcluster, "API String"=w185:string, "Cluster Data (dup)"=w186:T5)  [unwired: 7 in]
      }
      frame "Data: Set Configuration" {
        n52 = call "Convert API String Arguments to Data.vim"("Reference Type"=w192, "API String"=w193) -> ("error out"=w190:errorcluster, "Data"=w191:T5)  [unwired: 6 in]
      }
      frame "Data: Update Indicators" {
      }
      frame "Data: Cleanup" {
        # "#CSM \"Data: Cleanup\"\nCleanup any data and references, here.\n(this is called automatically, by the Macro: Exit)"
        n53 = Unbundle By Name(w200) -> ("Core.Current VI Reference"=w203:refnum<vi>)
        n54 = Close Reference(reference=w203, error in (no error)=w202) -> (error out=w201:errorcluster)
        n55 = call <vilib>:"Add State(s) to Queue__JKI_lib_State_Machine.vi"("State(s) in (\"\")"=w205) -> ("States Out"=w204:string)  [unwired: 14 in]
      }
      frame "---------- Macro ----------" {
        # "#CSM \"Category Seperator\"\nDo not put any code in this frame."
        n56 = call <vilib>:"Add State(s) to Queue__JKI_lib_State_Machine.vi"("State(s) in (\"\")"=w210) -> ("States Out"=w209:string)  [unwired: 14 in]
      }
      frame "Macro: Initialize" {
        # "#CSM \"Macro: Initialize\"\nInitialization Macro (This is called once, when the VI starts)"
        n57 = call <vilib>:"Add State(s) to Queue__JKI_lib_State_Machine.vi"("State(s) in Front (\"\")"="Data: Initialize\nInitialize Core Data\nData: Update Indicators", "State(s) in (\"\")"=w216) -> ("States Out"=w215:string)  [unwired: 13 in]
      }
      frame "Macro: Exit" {
        # "#CSM \"Macro: Exit\"\nExit Macro (This is called once, when the VI exits)"
        n58 = call <vilib>:"Add State(s) to Queue__JKI_lib_State_Machine.vi"("State(s) in Front (\"\")"="Data: Cleanup\nExit", "State(s) in (\"\")"=w222) -> ("States Out"=w221:string)  [unwired: 13 in]
      }
      frame "---------- API ----------" {
        # "#CSM \"Category Seperator\"\nDo not put any code in this frame."
      }
      frame "Channels" {
        n59 = disable-structure "Diagram Disable Structure" shown="Enabled" {
          disable-tunnel: [w232 w235] -> w229
          disable-tunnel: w227 -> [_ w236]
          frame Disabled {
            n60 = Initialize Array("" ("element"), 4 ("dimension size")) -> (w232:string[])
          }
          frame Enabled {
            n61 = Unbundle By Name(w236) -> ("Channels"=w235:string[])
          }
        }
        n62 = call "Convert Data To API String Arguments.vim"("Data"=w229) -> ("API String"=w228:string)  [unwired: 7 in, 1 out]
      }
      frame "read" {
        # "#CSM API Example\nCopy/Rename this case for your own API"
        n63 = call "Convert API String Arguments to Data.vim"("Reference Type"=cluster{"Channel":string, "Num":i32} {"Channel"="ai/1", "Num"=1}, "API String"=w249) -> ("Data"=w247:cluster{"Channel":string, "Num":i32})  [unwired: 6 in, 1 out]
        n64 = Unbundle By Name(w247) -> ("Channel"=w238:string, "Num"=w246:i32)
        n65 = Unbundle By Name(w244) -> ("Channels"=w243:string[])
        n66 = To Lower Case(string=w243) -> (all lower case string=w241:string[])
        n67 = To Lower Case(string=w238) -> (all lower case string=w242:string)
        n68 = Search 1D Array(1D array=w241, element=w242) -> (index of element=w240:i32)  [unwired: 1 in]
        n69 = Greater Or Equal To 0?(x=w240) -> (x >= 0?=w239:bool)
        n70 = case shown="True" w239 {
          tunnel: w246 -> [_ w258]
          tunnel: [_ w256] -> w245
          tunnel: w238 -> [w253 _]
          tunnel: [w251 _] -> w237
          frame False {
            n71 = Format Into String(format string="Channel \"%s\" is not found", w253) -> (resulting string=w252:string)  [unwired: 2 in, 1 out]
            n72 = call <userlib>:"Build Error Cluster.vi"("String to Prepend to Source (\"\")"=w252, "Code"=-1 ("code")) -> ("error out"=w251:errorcluster)
          }
          frame True {
            n73 = for {
              N: w258 -> [_]
              tunnel: [w259] -> w257 mode=indexing
              n74 = Random Number (0-1)() -> (number: 0 to 1=w259:dbl)
            }
            n75 = call "Convert Data To API String Arguments.vim"("Data"=w257) -> ("API String"=w256:string)  [unwired: 7 in, 1 out]
          }
        }
      }
      frame "read(massdata)" {
        # "#CSM API Example\nCopy/Rename this case for your own API"
        n76 = call "Convert API String Arguments to Data.vim"("Reference Type"=cluster{"Channel":string, "Num":i32} {"Channel"="ai/1", "Num"=1}, "API String"=w272) -> ("Data"=w270:cluster{"Channel":string, "Num":i32})  [unwired: 6 in, 1 out]
        n77 = Unbundle By Name(w270) -> ("Channel"=w261:string, "Num"=w269:i32)
        n78 = Unbundle By Name(w267) -> ("Channels"=w266:string[])
        n79 = To Lower Case(string=w266) -> (all lower case string=w264:string[])
        n80 = To Lower Case(string=w261) -> (all lower case string=w265:string)
        n81 = Search 1D Array(1D array=w264, element=w265) -> (index of element=w263:i32)  [unwired: 1 in]
        n82 = Greater Or Equal To 0?(x=w263) -> (x >= 0?=w262:bool)
        n83 = case shown="True" w262 {
          tunnel: w269 -> [_ w282]
          tunnel: [_ w280] -> w268
          tunnel: w261 -> [w276 _]
          tunnel: [w274 w279] -> w260
          frame False {
            n84 = Format Into String(format string="Channel \"%s\" is not found", w276) -> (resulting string=w275:string)  [unwired: 2 in, 1 out]
            n85 = call <userlib>:"Build Error Cluster.vi"("String to Prepend to Source (\"\")"=w275, "Code"=-1 ("code")) -> ("error out"=w274:errorcluster)
          }
          frame True {
            n86 = for {
              N: w282 -> [_]
              tunnel: [w283] -> w281 mode=indexing
              n87 = Random Number (0-1)() -> (number: 0 to 1=w283:dbl)
            }
            n88 = call "CSM - Convert MassData to Argument.vim"("Data"=w281) -> ("error out"=w279:errorcluster, "MassData Argument"=w280:string)  [unwired: 7 in]
          }
        }
      }
      frame "read all" {
        w287 = 1  # Num
        # "#CSM API Example\nCopy/Rename this case for your own API"
        n89 = call "Convert API String Arguments to Data.vim"("Reference Type"=w287, "API String"=w290) -> ("Data"=w286:i32)  [unwired: 6 in, 1 out]
        n90 = Unbundle By Name(w285) -> ("Channels"=w284:string[])
        n91 = for {
          tunnel: [w294] -> w289 mode=indexing
          tunnel: w286 -> [w293]
          tunnel: w284 -> [_] mode=indexing
          n92 = for {
            N: w293 -> [_]
            tunnel: [w295] -> w294 mode=indexing
            n93 = Random Number (0-1)() -> (number: 0 to 1=w295:dbl)
          }
        }
        n94 = call "Convert Data To API String Arguments.vim"("Data"=w289) -> ("API String"=w288:string)  [unwired: 7 in, 1 out]
      }
      frame "---------- DoSth ----------" {
        # "#CSM \"Category Seperator\"\nDo not put any code in this frame."
        n95 = call <vilib>:"Add State(s) to Queue__JKI_lib_State_Machine.vi"("State(s) in (\"\")"=w300) -> ("States Out"=w299:string)  [unwired: 14 in]
      }
      frame "DoSth: DoA" {
        # "#CSM \"Internal State\"\nThis category is used for holding internal states"
        n96 = call <vilib>:"Add State(s) to Queue__JKI_lib_State_Machine.vi"("State(s) in (\"\")"=w305) -> ("States Out"=w304:string)  [unwired: 14 in]
      }
      frame "DoSth: DoB" {
        # "#CSM \"Internal State\"\nThis category is used for holding internal states"
        n97 = call <vilib>:"Add State(s) to Queue__JKI_lib_State_Machine.vi"("State(s) in (\"\")"=w310) -> ("States Out"=w309:string)  [unwired: 14 in]
      }
    }
  }
